vi "Packet Recorder Mode.vi"() -> (0 "Reading?":bool, 1 "Writing?":bool)   [LabVIEW 2012, in "Packet Recorder.lvlib"]
uses:
  Packet Recorder.lvlib
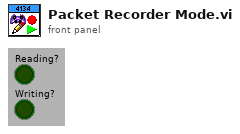
[diagram p1: front panel]
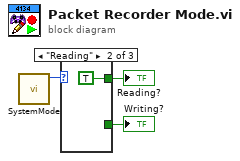
[diagram p0: block diagram]
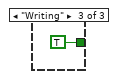
[diagram p3: hidden frame]
diagram:
  n1 = call "SystemMode.vi"() -> ("Mode"=w3:enum16{"Off", "Reading", "Writing"})  [unwired: 11 in]
  n2 = case shown="\"Reading\"" w3 {
    tunnel: [_ TRUE _] -> w2
    tunnel: [_ _ TRUE] -> w1
    frame "Off", Default {
    }
    frame "Reading" {
    }
    frame "Writing" {
    }
  }
  "Reading?" <- w2
  "Writing?" <- w1
